vi "Get SMO Database Paths.vi"(5 "getAll Cluster":variant, 7 "Default Paths":string, 8 "error in (no error)":errorcluster, 11 "instrument.OptiCool in":refnum<class "instrument.OptiCool.lvclass">) -> (0 "error out":errorcluster, 2 "Paths":string, 3 "instrument.OptiCool out":refnum<class "instrument.OptiCool.lvclass">)   [LabVIEW 2019, in "instrument.OptiCool.lvclass"]
uses:
  instrument.OptiCool.lvclass
  instrument.PPMS/Typedefs/PPMS.getAll--cluster.ctl
  instrument.PPMS/instrument.PPMS.lvclass
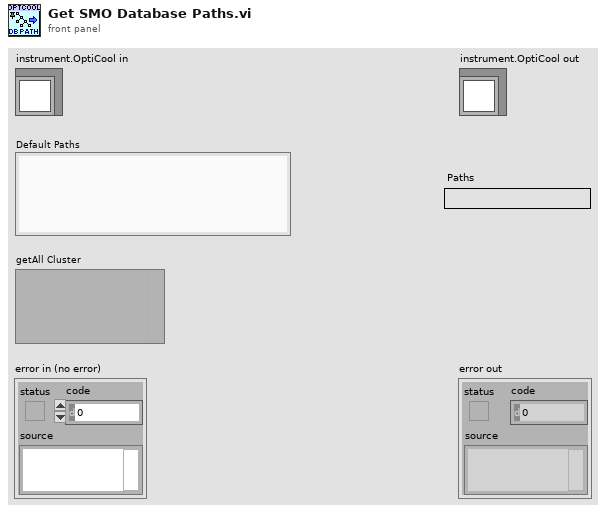
[diagram p1: front panel]
types:
  T1 = typedef "instrument.PPMS.lvclass/PPMS.getAll--cluster.ctl" = cluster{"Chamber Status":string, "Helium Level":dbl, "Temperature":dbl, "Temperature Status":string, "Magnetic Field":dbl, "Magnet Status":string, "Position":dbl}
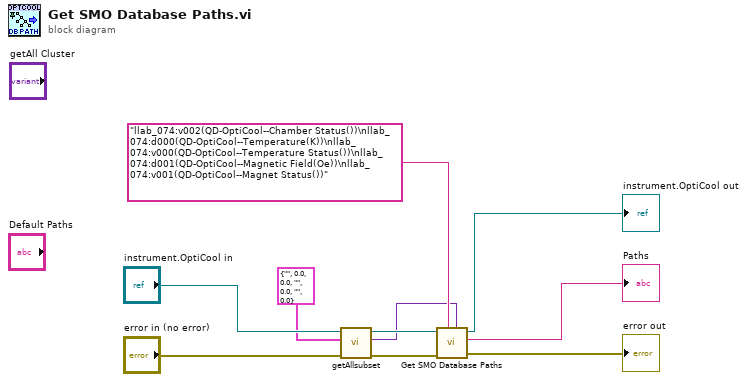
[diagram p0: block diagram]
diagram:
  n1 = call-dynamic "getAllsubset.vi"("error in (no error)"="error in (no error)", "getAll"=T1 {"Chamber Status"="", "Helium Level"=0.0, "Temperature"=0.0, "Temperature Status"="", "Magnetic Field"=0.0, "Magnet Status"="", "Position"=0.0}, "instrument.OptiCool in"="instrument.OptiCool in") -> ("error out"=w3:errorcluster, "output cluster"=w2:variant, "instrument.OptiCool out"=w4:refnum<class "instrument.OptiCool.lvclass">)  [unwired: 6 in]
  n2 = call-parent "Get SMO Database Paths.vi"("getAll Cluster"=w2, "Default Paths"="llab_074:v002(QD-OptiCool--Chamber Status())\nllab_074:d000(QD-OptiCool--Temperature(K))\nllab_074:v000(QD-OptiCool--Temperature Status())\nllab_074:d001(QD-OptiCool--Magnetic Field(Oe))\nllab_074:v001(QD-OptiCool--Magnet Status())" ("Paths"), "error in (no error)"=w3, "instrument.PPMS in"=w4) -> ("error out"=→"error out":errorcluster, "Paths"=→"Paths":string, "instrument.PPMS out"=→"instrument.OptiCool out":refnum<class "instrument.OptiCool.lvclass">)  [unwired: 5 in]
